vi "GUI.vi"() -> ()   [LabVIEW 2019]
uses:
  song-structure.ctl
  Project Parameters.ctl
  statemachine.ctl
  <vilib>/Platform/TimedLoop/XDataNode/timing_clust.ctl
  <vilib>/Platform/TimedLoop/XDataNode/nitl_modes.ctl
  <vilib>/Platform/TimedLoop/XDataNode/wakeup.ctl
  53cbb8c8-3a7e-4936-be36-e47a8a17bf59.vi
  <vilib>/numeric/Random Number (Range) I64.vi
  <vilib>/numeric/sub_Random U32.vi
  <vilib>/Utility/file.llb/Read Delimited Spreadsheet (string).vi
  <vilib>/platform/TimedLoop/XDataNode/XDataNode.xnode
  Windows/System32/winmm.dll
  <vilib>/Platform/TimedLoop/XDataNode/XDNodeRunTimeDep.lvlib
panel:
  out "Reaperproject folder path":path
  out "Progression":i32(knob) scale=0.0..10.0
  out "MIDI-notes":string[](array[string])
  out "Chord MIDI-values":string[][](array[string])
  out "Chord Frequencies":dbl[][][](array[numeric])
  out "Project Detail":T1
  out "Reaper Note":string
  in  "Exit":bool
  in  "Tab Control":T2(tab)
  in  "Guitarscale":bool
  out "Note 11":string
  out "Note 8":string
  out "Note 6":string
  out "Note 4":string
  out "Note 1":string
  out "Theme":string
  in  "Project name":string="Sett inn prosjektnavn her"
  out "Instruments":string[][](array[string])
  out "Special Musical Challenge":string
  out "Root":string
  out "Note 10":string
  out "Note 9":string
  out "Note 7":string
  out "Note 5":string
  out "Note 3":string
  out "Note 2":string
  out "Notes in Scale":bool[](array[boolean])
  in  "Låst BPM":i32=120
  in  "Lås BPM":bool
  out "Timesignature":string
  out "Tempo":i32
  in  "Language (H/B)":enum32{"Item 0", "Item 1"}(radio)
  in  "Initiate":bool
  out "Scale":string
  out "Key":string
  in  "Scale Categories":T3={"Minor"=TRUE, "Major"=TRUE, "Symmetric"=FALSE, "Pentatonic"=FALSE, "Bebop"=FALSE, "Blues"=FALSE, "Harmonic"=FALSE, "Exotic"=FALSE, "Misc."=FALSE}
  out "Length":string
  in  "Timesignatures":T4={"Commontime"=TRUE, "Simple"=TRUE, "Compound"=FALSE, "Complex"=FALSE}
  out "Song Structure":string[](array[string])
  in  "Reap":bool
  out "Chords":string[][](array[string])
  out "Notes":string[](array[string])
  in  "Grunntone":bool
  in  "Metronom":bool
  in  "Stop Music":bool
  in  "Ordinære\nakkorder":bool
  in  "MIDI-fil":bool
  in  "Play":bool
  in  "Create Chord Progression":bool
  out "Handler":i32
  out "Romans":string[](array[string])
  out "Chordnames":string[](array[string])
  out "Chord active":bool[](array[boolean])
  in  "Instrument":i32(listbox)
  in  "Volume":i32(slide)=99 scale=0.0..127.0
  in  "Fastest BPM":i32=170
  in  "Slowest BPM":i32=50
  in  "Song structure":T5={"Intro %"=50.0, "Bridge %"=50.0, "Solo %"=50.0, "Outro %"=50.0, "Min # Vers"=2, "Max # Vers"=5, "Min # Refreng"=2, "Max # Refreng"=4, "Measure per phrase"=4, "Phrase per part"=4} {"Outro %" format="%#_13g"; "Solo %" format="%#_13g"; "Bridge %" format="%#_13g"; "Intro %" format="%#_13g"}
  in  "CPU timing":u32=50
  in  "# instruments":i32=8
  in  "# Themes":i32=3
  out "Path of the program":path
  # "(Pick 5)"
  # "This will generate a folder! with 2 files:\n- List of chords\n- Reaper project"
  # "Available chords in the given key and scale"
  # "Chord Progression"
  # "The chord progression is generated based on the parameters from the project tab. The parameters are not altered."
  # "Settings of creation"
  # "*Not all scales work equally"
  # "Settings"
  # "I was unable to alter some of the text above without doing too much work. \"Refreng\" = Chorus, \"Vers\" = Verse. Hopefully you'll survive."
  # "About the software"
  # "Features I considered"
  # "This software was created to learn more about state machines, as well as create a software that challenges my musical/ recording skills. It's main function is to generate a musical recording challenge, by listing parameters for the user to comply to. This way the musician can focus on recording and the creative parts, instead of waiting for an idea."
  # "- Random project name\n- Jam function, without using Reaper\n-"
  # "Problems"
  # "Reaper project"
  # "At the moment the software will only have full functionality in administrative mode (Windows settings). This is only related to running a .exe-file. Avoid always having to choosing this mode by:\n1. Rightclicking the \"usic.exe\"-file.\n2. Go to settings.\n3. Open the tab \"Compatibily\".\n4.  Check the \"Run this program as administrator\" and hit OK \n\nThese names were directly translated, you experience may vary."
  # "Hvordan bruker man programmet"
  # "Under the \"Project\" tab you can generate random song parameters. Possible tempo, timesignatures and scales are selected before generating.\n\nIn the Chords tab you'll find chords that should fit the key and scale mentioned in the project tab.\n\nIn the Progression tab you can generate a chord progression that might be suitable for the given scale. Some chords and scales are more problematic. I therefore advice that you keep generating progressions and altering the settings of creation; untill you're satified with the result. The progression can then be put in stone by generating a MIDI file.\n\nThe settings tab is for thinkering with the odds of the generator."
  # "Other problems"
  # "The program crashes if you abort the creation of the reaper project folder."
  # "Musical Improv Exercise"
  # "Regler underveis"
  # "Spillet fungerer som \"ett ord om gangen eventyr\". Istedet for at hver deltaker legger til et ord, legger man til et musikalsk uttrykk.\n\n1. Den startende deltakeren starter et Reaper-prosjekt ved hjelp av dette programmet, og spiller inn ett opptak. Hvor langt opptaket er velger deltakeren selv.\n2. Prosjektet lagres og neste man får beskjed om at det er hans tur.\n3. Neste man spiller inn ett nytt opptak, og utfører punkt 2.\n\nPunkt 2 og 3 gjenntas til prosjektets krav er nådd og alle føler prosjektet er ferdig nok til miksing.\n\nStartende deltaker for i oppgave å starte miksingen, og når man føler seg ferdig blir prosjektet sendt til neste man. Dette gjentas til alle har deltatt i miksingen, miksen er nå klar for mastering.\n\nMastering fungerer på samme måte som miksing."
  # "- Bordet fanger; det vil si at man ikke kan slette tidligere endringer. Hverken sine egne innspillinger, og tillagte effekter; eller andre innspillinger. og tillagte effekter\n- Hver runde med innspilling er det mulighet for å legge effekter på spor, men ikke fjerne.\n- Det er ikke tillat å endre på prosjektparameterene oppgitt i Reaper-notatet. Altså der som genereres av startende deltaker.\n- Hver låt må ha vokal, men foruten det kan man fjerne opptil 3 instrumenter av de genererte 8.\n- Tema er opp til hver enkelt deltaker å tolke.\n- Bruker man plugins som ikke er inkludert i Reaper, må det lages et hjelpespor med effekten inebygget i sporet. Slik at man slipper plugins-en."
  # "Deling av prosjekt"
  # "Formålet"
  # "Prosjektet deles via avtalt plattform.\nHver nøye på å se over plugins."
  # "Hensikten med programmet og øvelsen er mengdetrening, eksponering og å ha det gøy. Derfor skal man ikke bruke timer på den perfekte overgangen, miksingen eller teksten. Om man ønsker en standard for musikalsk kvalitet og dybde, se til band som Bloodhound gang, Bare Egil Band,  Hurra Torpedo mm."
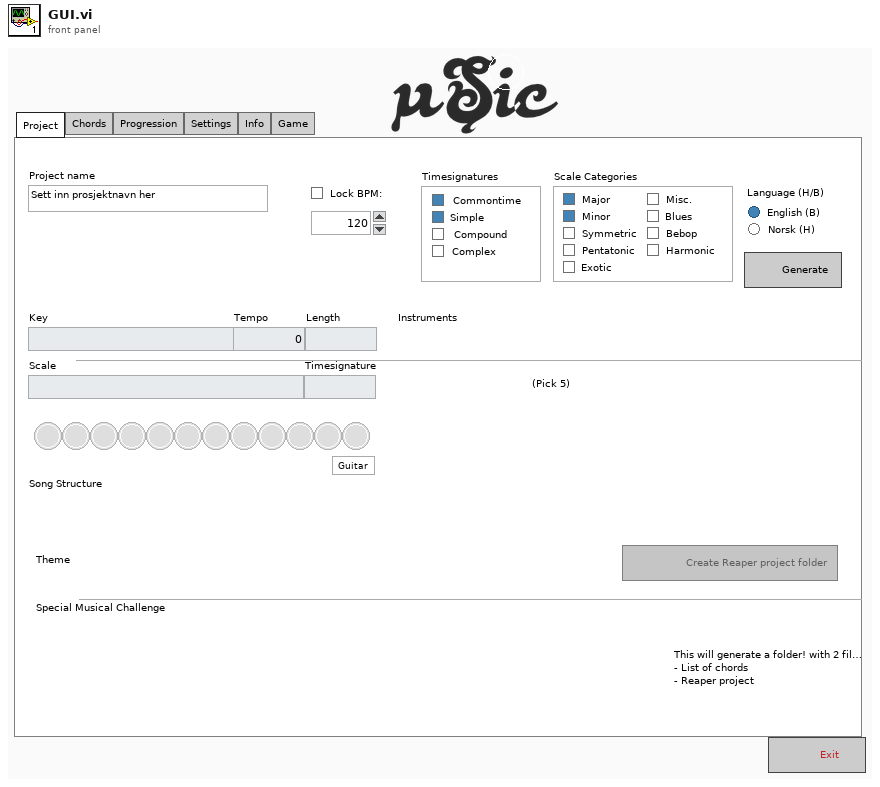
[diagram p1: front panel]
types:
  T1 = typedef "Project Parameters.ctl" = cluster{"Song Structure":string[], "Song Length":string, "Timesignature":string, "Key":string, "Scale":string, "Bpm":i32, "Tema":string, "Prosjekt tittel":string, "Challenge":string, "Instruments":string[]}
  T2 = enum32{"Project", "Chords", "Progression", "Settings", "Info", "Game"}
  T3 = cluster{"Minor":bool, "Major":bool, "Symmetric":bool, "Pentatonic":bool, "Bebop":bool, "Blues":bool, "Harmonic":bool, "Exotic":bool, "Misc.":bool}
  T4 = cluster{"Commontime":bool, "Simple":bool, "Compound":bool, "Complex":bool}
  T5 = typedef "song-structure.ctl" = cluster{"Intro %":dbl, "Bridge %":dbl, "Solo %":dbl, "Outro %":dbl, "Min # Vers":i32, "Max # Vers":i32, "Min # Refreng":i32, "Max # Refreng":i32, "Measure per phrase":i32, "Phrase per part":i32}
  T6 = typedef "statemachine.ctl" = enum16{"Boot", "Wait for Event", "Play music", "Stop music", "Shut down", "MIDI-file shutdown"}
  T7 = enum16{"open", "replace", "create", "open or create", "replace or create", "replace or create with confirmation"}
  T8 = enum8{"Enabled", "Disabled", "Disabled and Grayed Out"}
  T9 = typedef "XDNodeRunTimeDep.lvlib/timing_clust.ctl" = cluster{"Expected End [f-1]":u64, "Actual End [f-1]":u64, "Finished Late? [f-1]":bool, "Expected End [i-1]":u64, "Actual End [i-1]":u64, "Finished Late? [i-1]":bool, "Expected Start [i]":u64, "Actual Start [i]":u64, "Expected Start [f]":u64, "Actual Start [f]":u64, "Source Name":string, "Structure Name":string, "Period":i64, "Deadline":i64, "Offset":i64, "Start":i64, "Priority":i32, "Timeout":i32, "Mode":T10, "Wakeup Reason":T11, "Error":errorcluster, "Source Type":string, "Secondary Source Type":string, "Global End Time":u64, "Global Start Time":u64, "Frame Duration":u64, "Iteration Duration":u64, "Assigned CPU":i32, "I/O Scan Engine Mode":u32}
  T10 = typedef "XDNodeRunTimeDep.lvlib/nitl_modes.ctl" = enum32{"No Change", "Process missed periods, maintain original phase", "Discard missed periods, maintain original phase", "Process missed periods, ignore original phase", "Discard missed periods, ignore original phase"}
  T11 = typedef "XDNodeRunTimeDep.lvlib/wakeup.ctl" = enum32{"Normal", "Aborted", "Asynchronous wakeup", "Timing source error", "Timed loop error", "Timeout"}
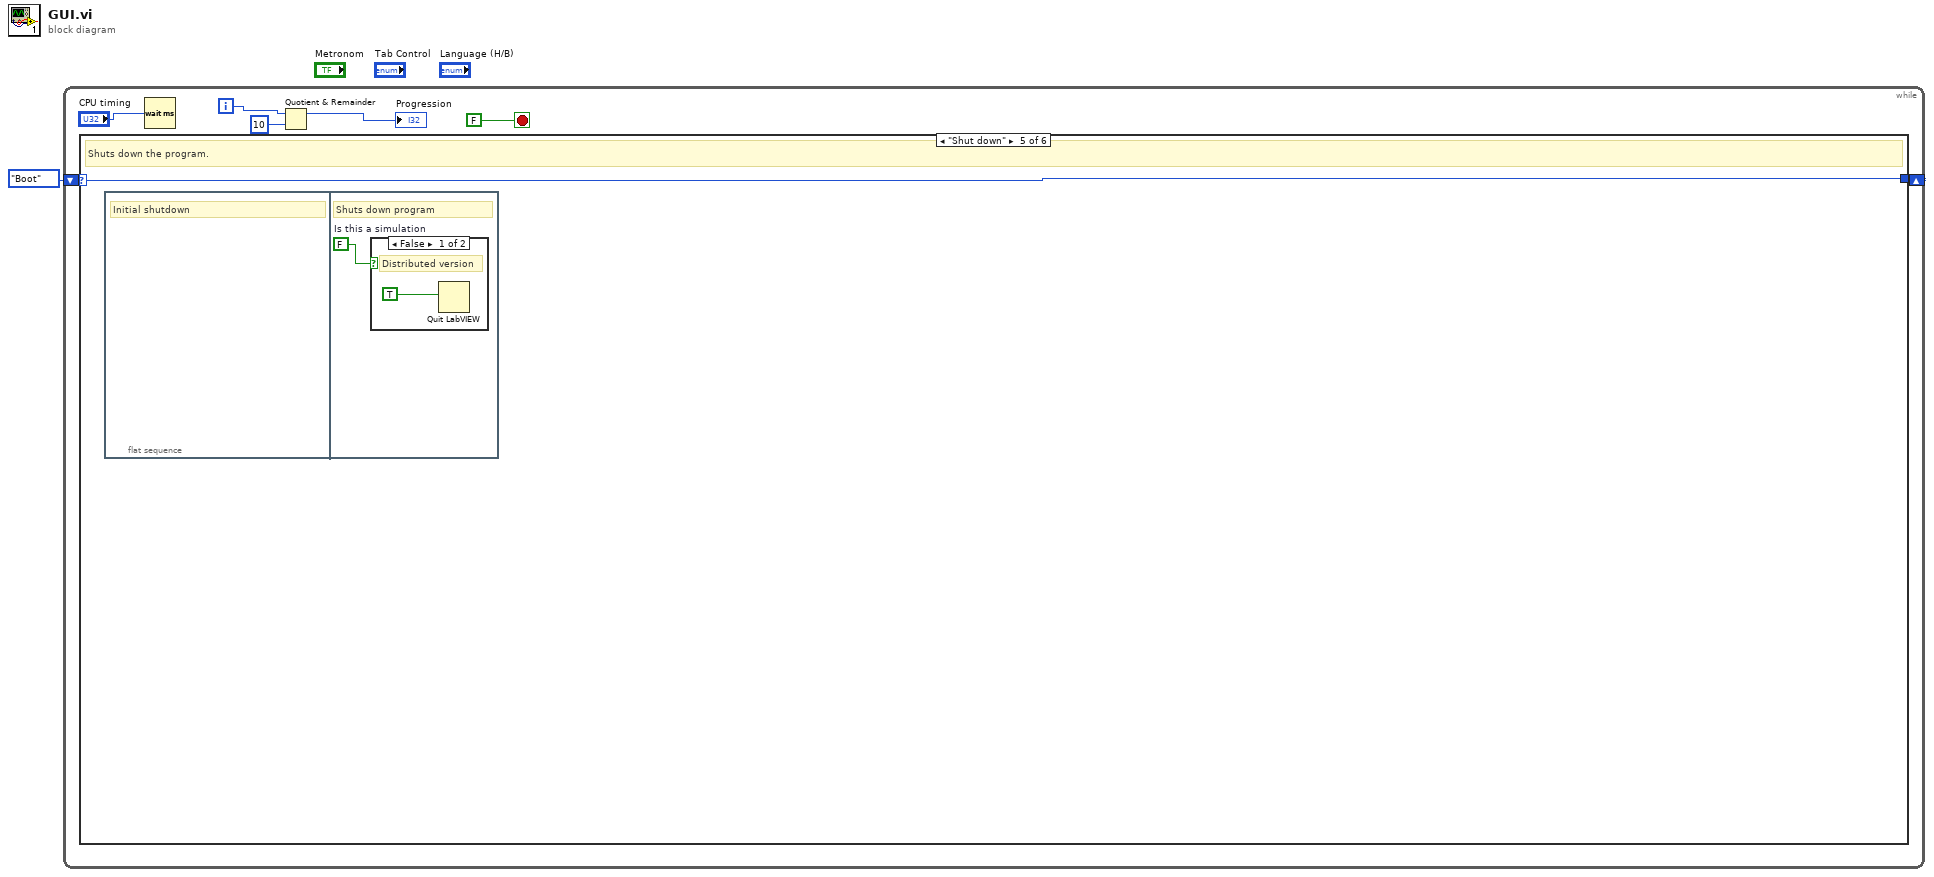
[diagram p0: block diagram]
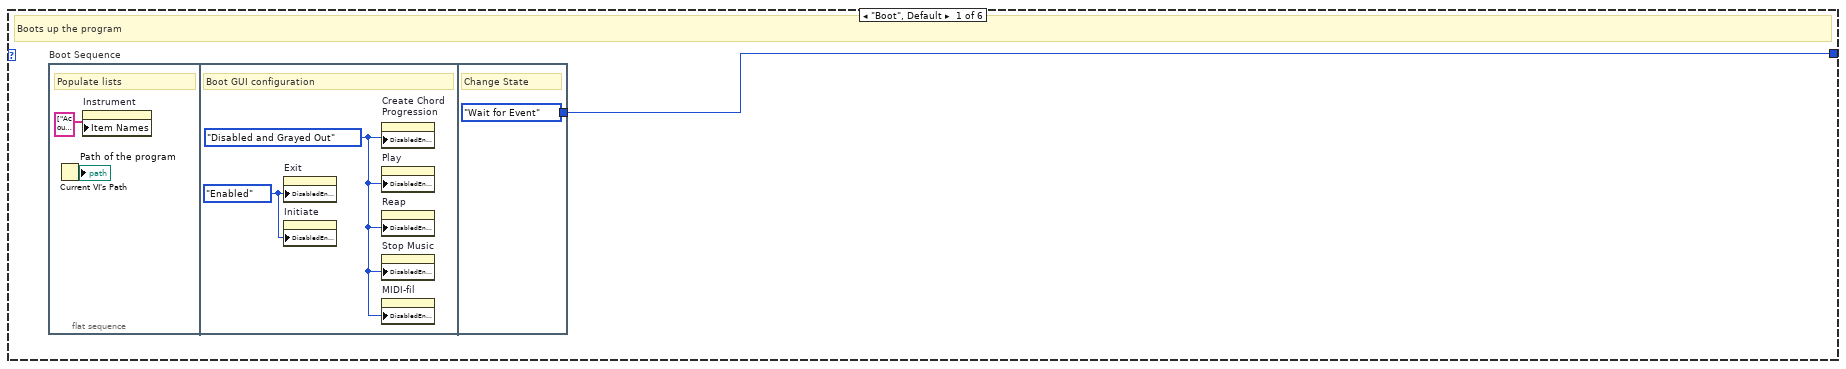
[diagram p2: hidden frame]
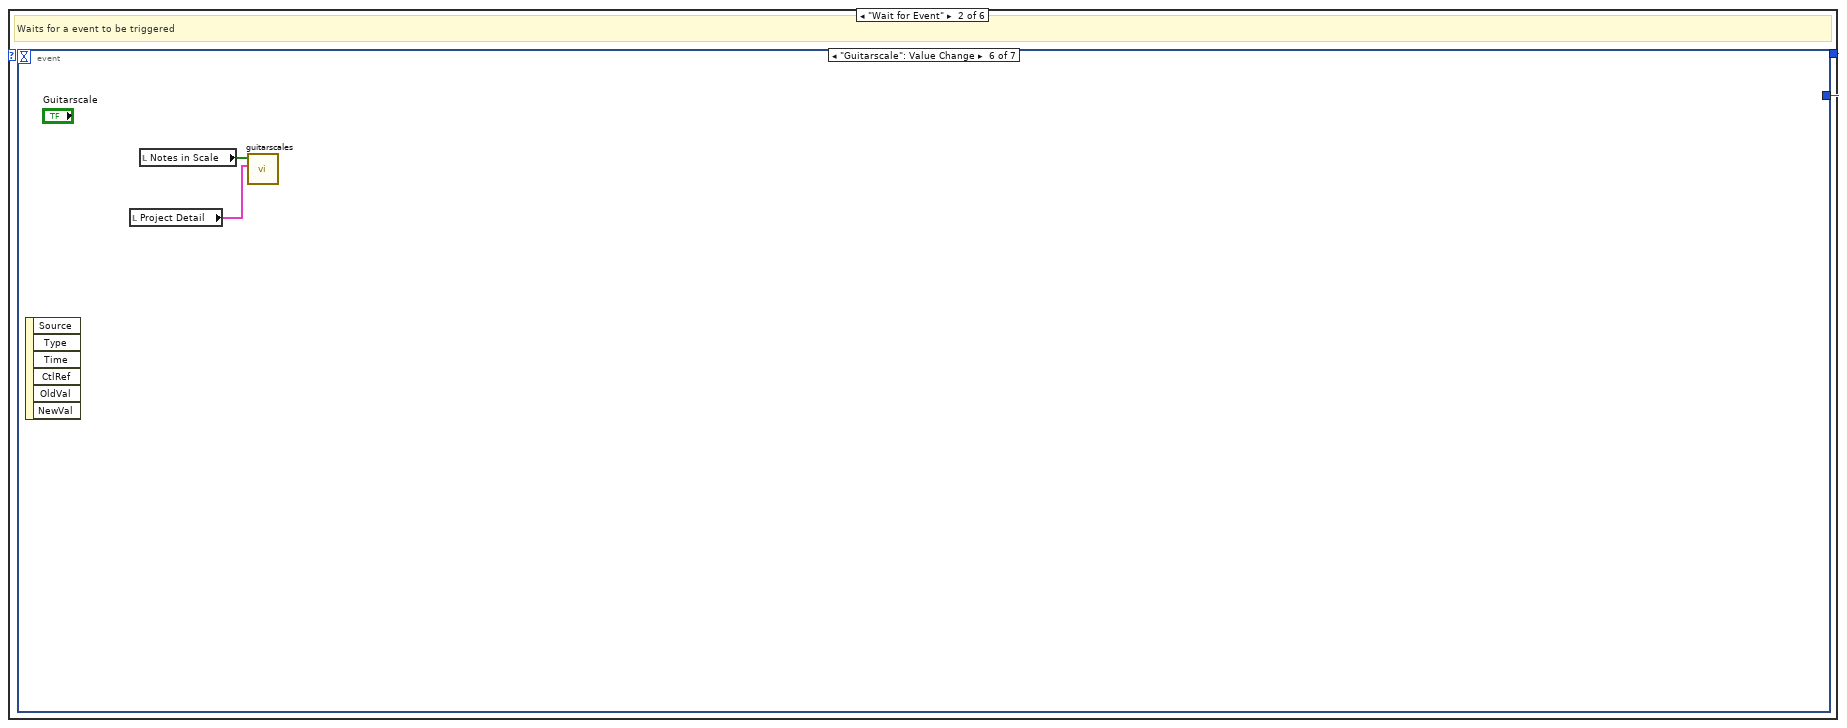
[diagram p3: hidden frame]
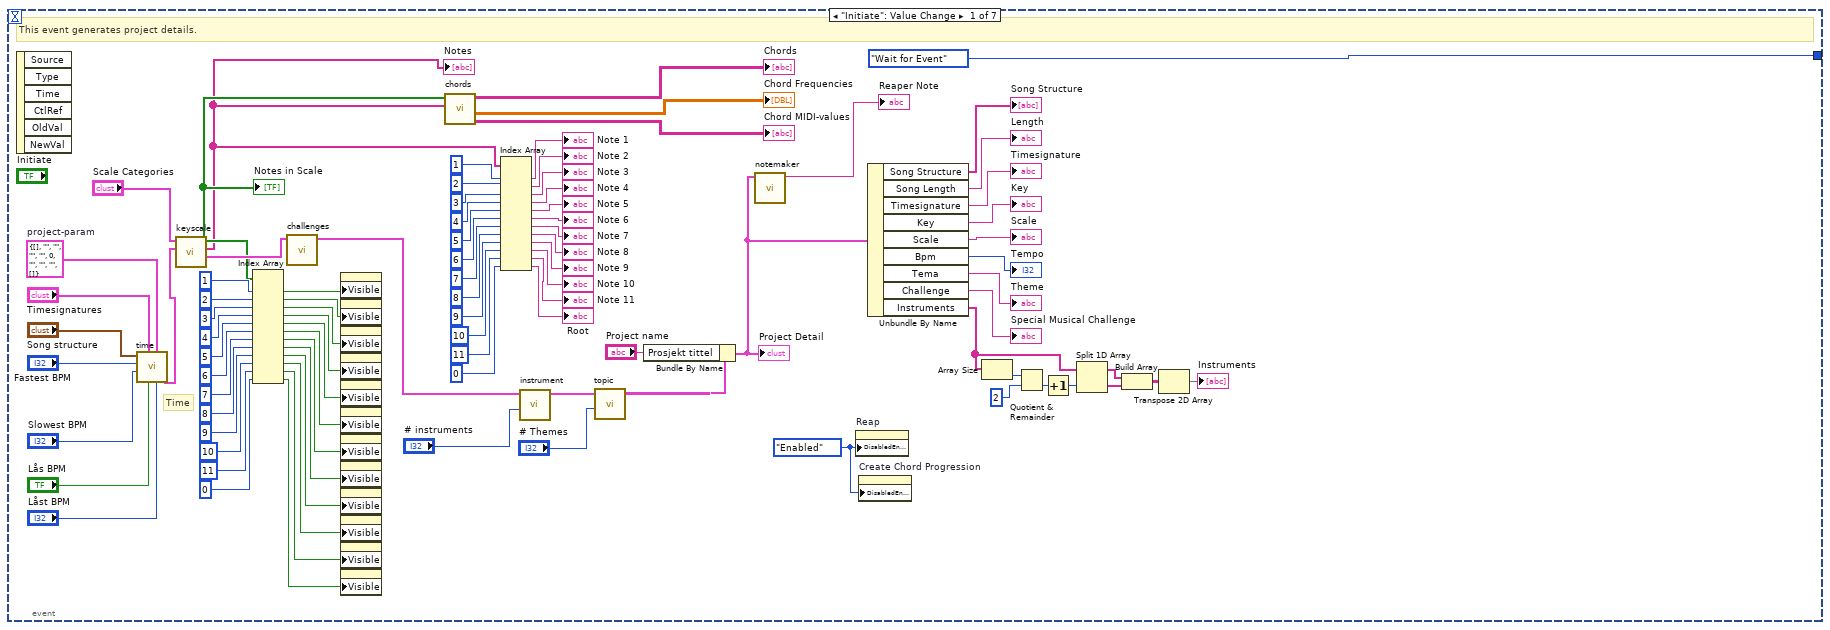
[diagram p4: hidden frame]
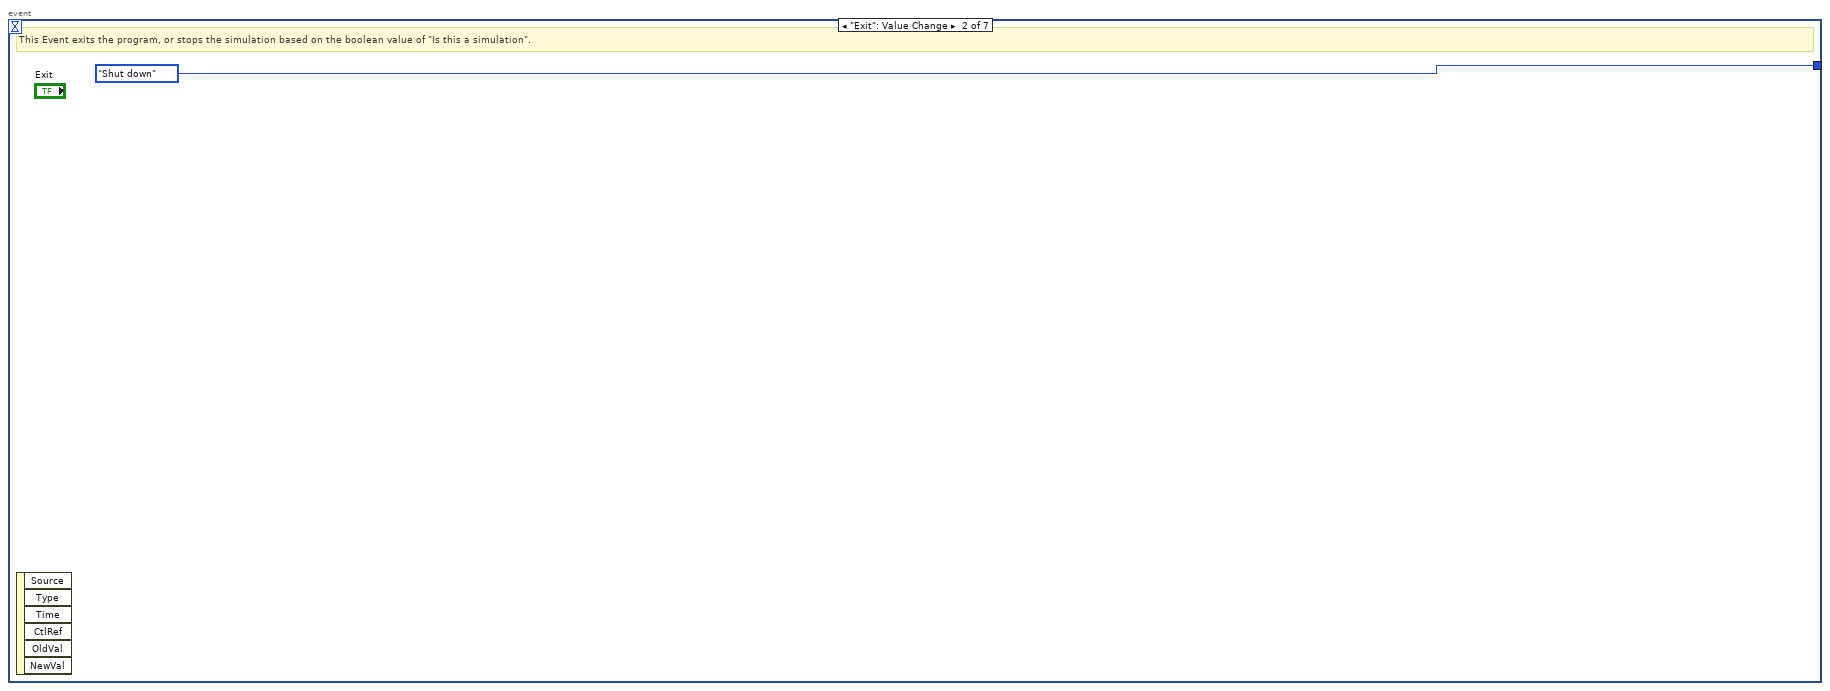
[diagram p5: hidden frame]
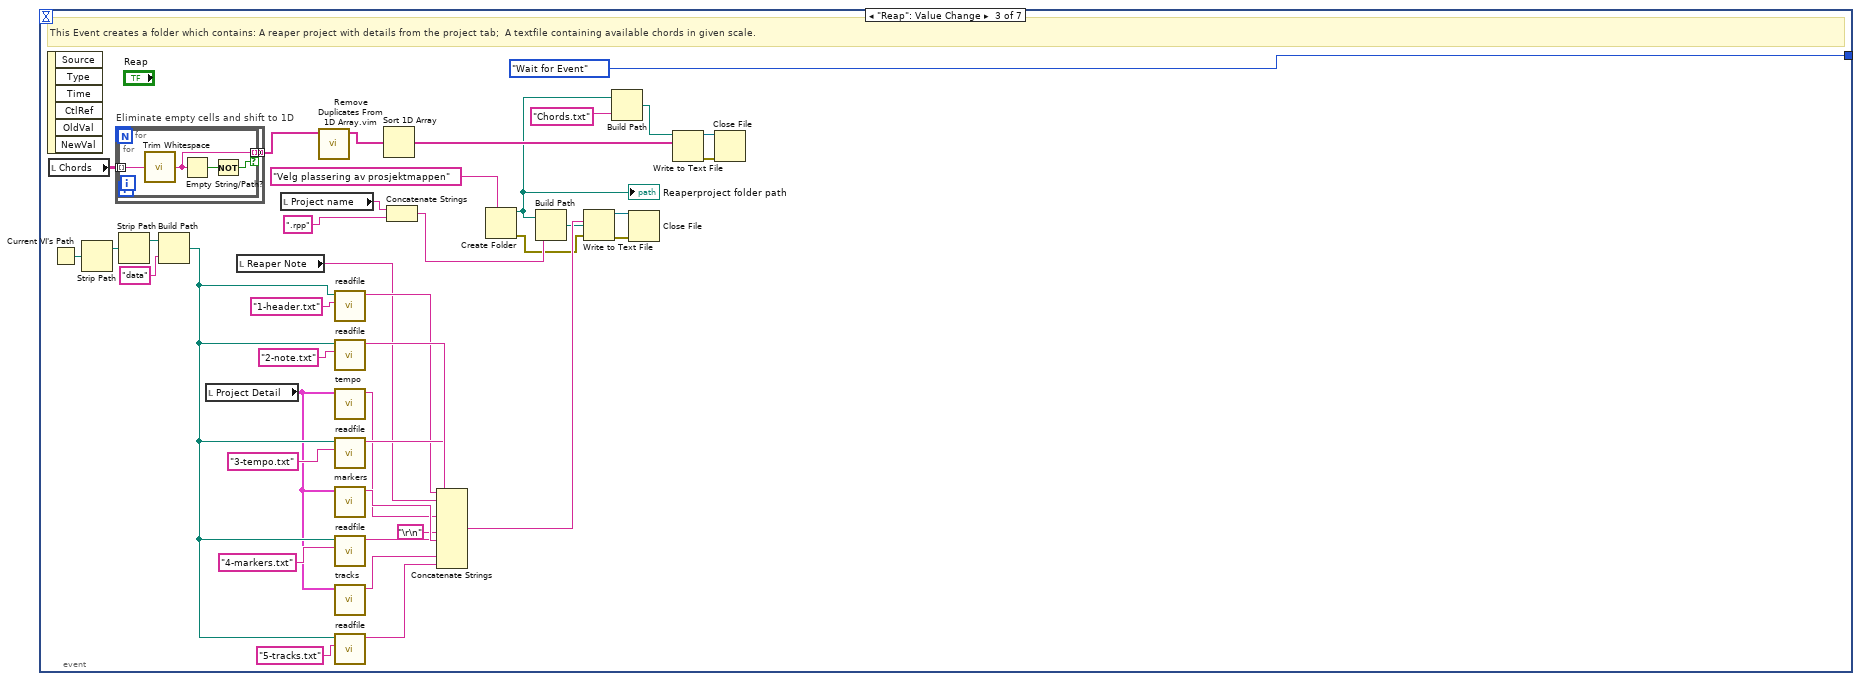
[diagram p6: hidden frame]
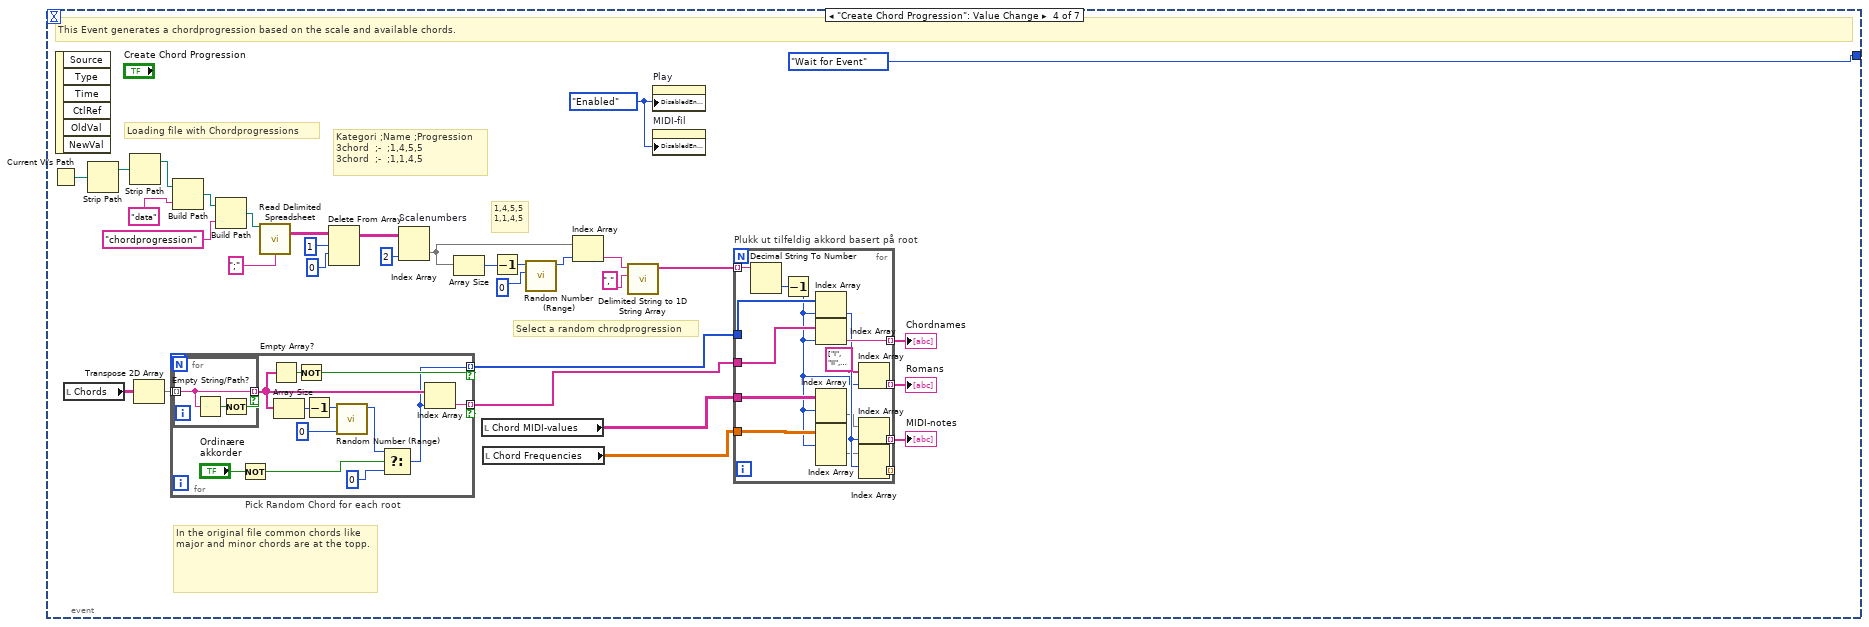
[diagram p7: hidden frame]
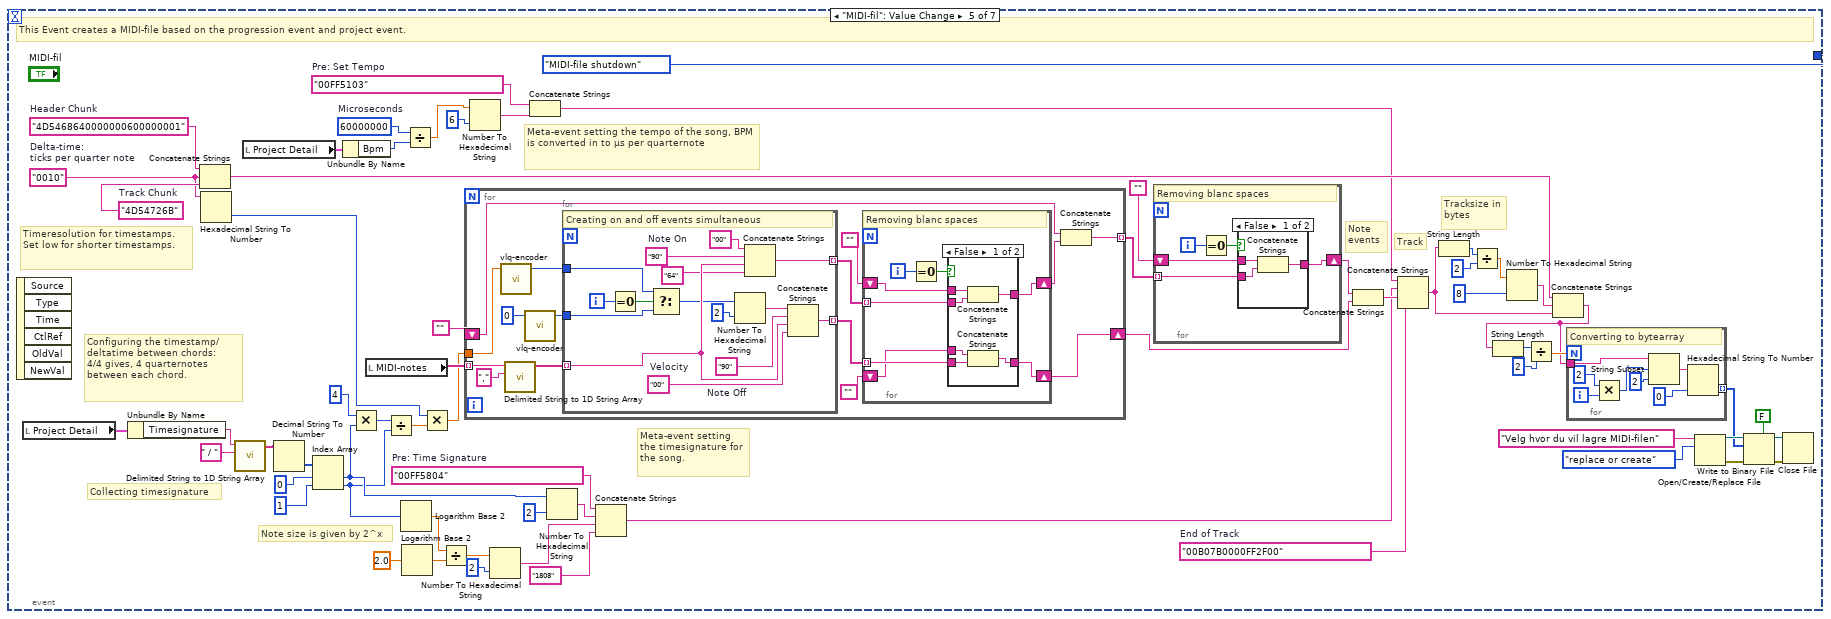
[diagram p8: hidden frame]
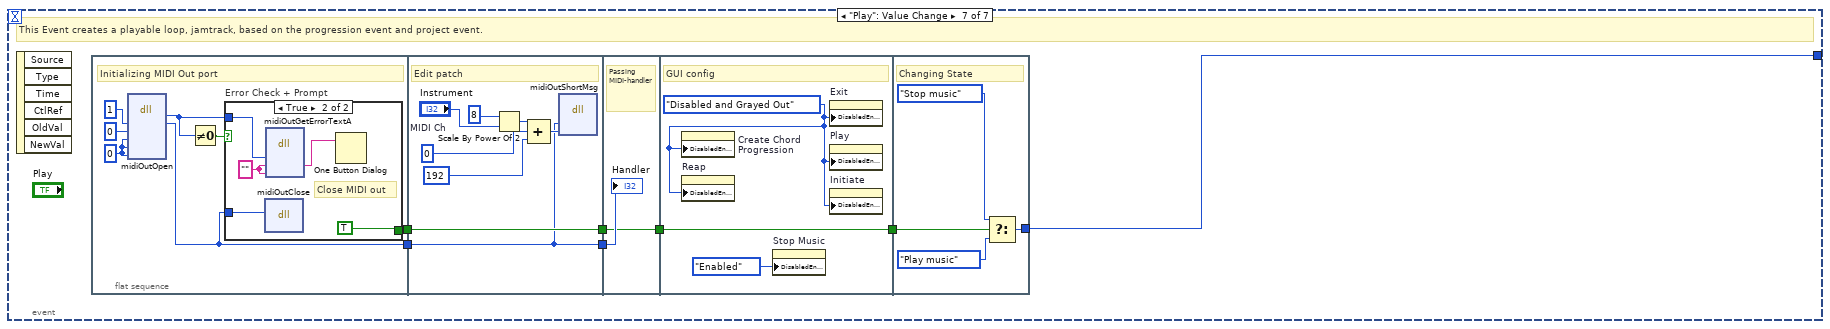
[diagram p11: hidden frame]
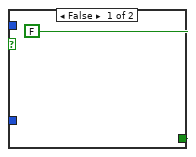
[diagram p12: hidden frame]
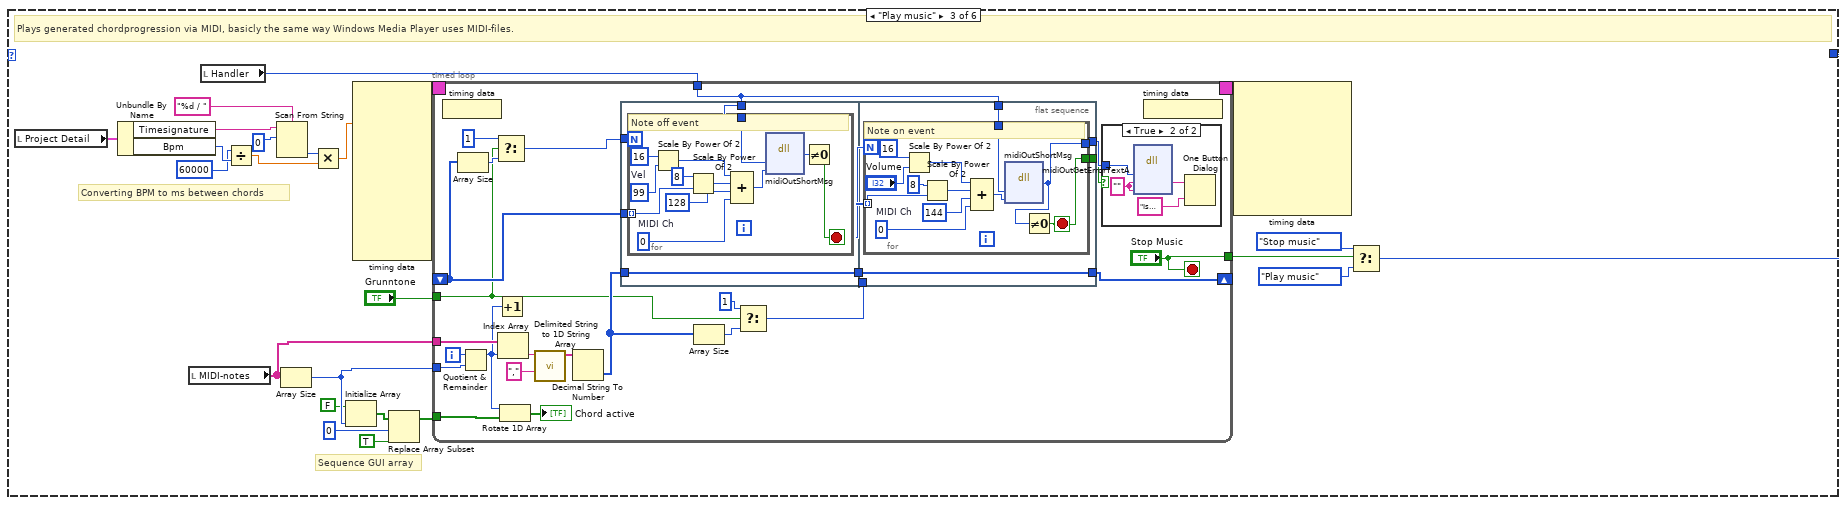
[diagram p13: hidden frame]
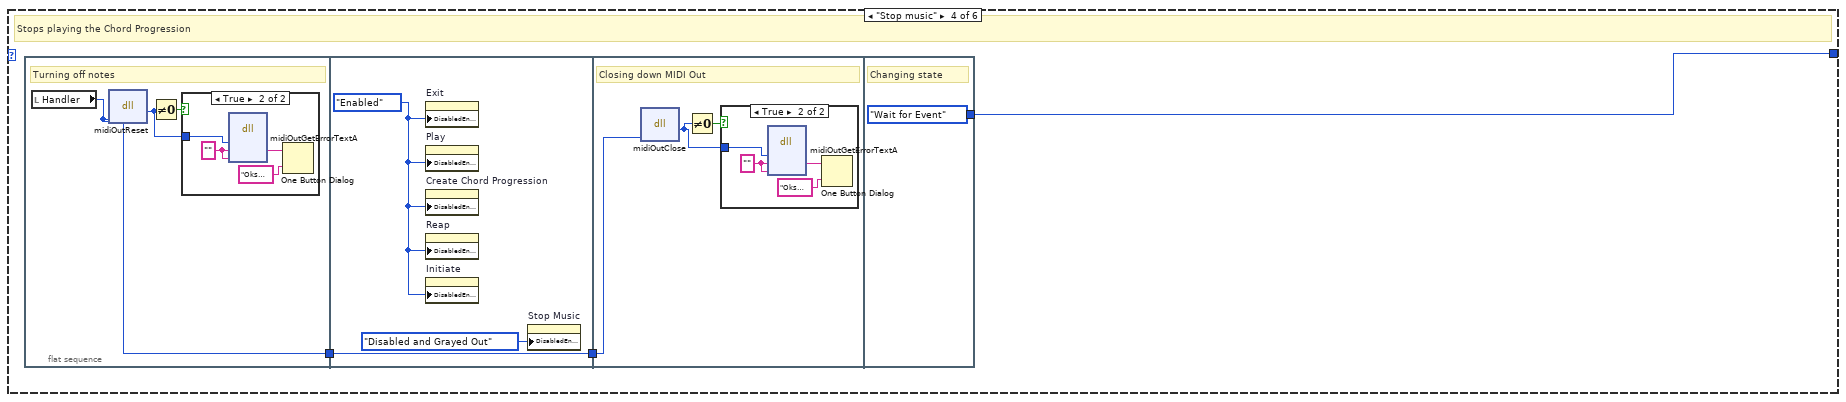
[diagram p15: hidden frame]
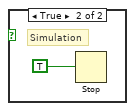
[diagram p18: hidden frame]
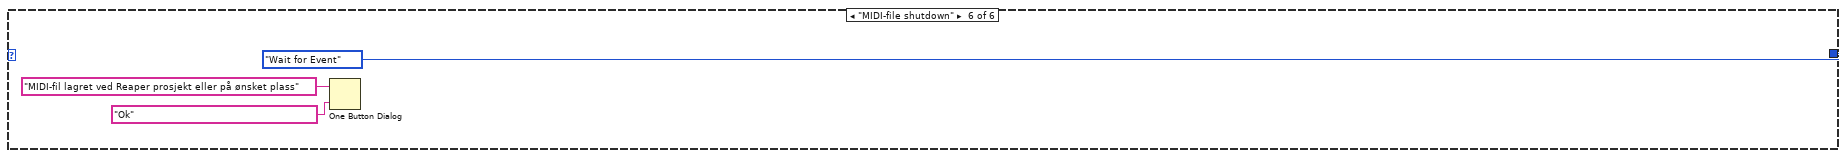
[diagram p19: hidden frame]
diagram:
  n1 = while {
    shift-right: [w2] -> _
    shift-left: statemachine."Boot" -> [w6]
    i -> [w5]
    stop <- FALSE stop-if-true
    n2 = case shown="\"Shut down\"" w6 {
      selector: w6 -> [_ _ _ _ w494 _]
      tunnel: [w9 w15 w403 w475 w494 statemachine."Wait for Event"] -> w2
      frame "Boot", Default {
        # "Boots up the program"
        n3 = flat-sequence "Boot Sequence" {
          tunnel: [statemachine."Wait for Event"] -> w9
          frame #0 {
            # "Populate lists"
            n4 = Current VI's Path() -> (path=→"Path of the program":path)
            n5 = property on="Instrument" class="LstBox (strict)"("Item Names"=string[] ["Acoustic Grand ", "Bright Acoustic ", "Electric Grand ", "Honky-tonk ", "Electric Piano I ", "Electric Piano 2 ", "Harpsichord ", "Clav ", "Perc Celesta ", "Perc Glockenspiel ", "Perc Music Box ", "Perc Vibraphone ", "Perc Marimba ", "Perc Xylophone ", "Perc Tubular Bells ", "perc Dulcimer ", "Drawbar Organ ", "Percussive Organ ", "Rock Organ ", "Church Organ ", "Reed Organ ", "Accordian ", "Harmonica ", "Tango Accordian ", "Acoustic Guitar (nylon) ", "Acoustic Guitar (steel) ", "Electric Guitar (jazz) ", "Electric Guitar (clean) ", "Electric Guitar (muted) ", "Overdriven Guitar ", "Distortion Guitar ", "Guitar Harmonics ", "Acoustic Bass ", "Electric Bass (finger) ", "Electric Bass (pick) ", "Fretless Bass ", "Slap Bass 1 ", "Slap Bass 2 ", "Synth Bass I ", "Synth Bass 2 ", "Violin ", "Viola ", "Cello ", "Contrabass ", "Tremolo Strings ", "Pizzicato Strings ", "Orchestral Strings ", "Timpani ", "String Ensemble 1 ", "String Ensemble 2 ", "Synth Strings I ", "Synth Strings 2 ", "Choir Aahs ", "Voice Oohs ", "Synth Voice ", "Orchestra Hit ", "Trumpet ", "Trombone ", "Tuba ", "Muted Trumpet ", "French Horn ", "Brass Section ", "Synth Brass I ", "Synth Brass 2 ", "Soprano Saxophone ", "Alto Saxophone ", "Tenor Saxophone ", "Baritone Saxophone ", "Oboe ", "English Horn ", "Bassoon ", "Clarinet ", "Piccolo ", "Flute ", "Recorder ", "Pan Flute ", "Blown Bottle ", "Shakuhachi ", "Whistle ", "Ocarina ", "Lead Lead 1 (square) ", "Lead Lead 2 (sawtooth) ", "Lead Lead 3 (calliope) ", "Lead Lead 4 (chiff) ", "Lead Lead 5 (charang) ", "Lead Lead 6 (voice) ", "Lead Lead 7 (fifths) ", "Lead Lead 8 (bass + lead) ", "Pad Pad 1 (new age) ", "Pad Pad 2 (warm) ", "Pad Pad 3 (polysynth) ", "Pad Pad 4 (choir) ", "Pad Pad 5 (bowed) ", "Pad Pad 6 (metallic) ", "Pad Pad 7 (halo) ", "Pad Pad 8 (sweep) ", "FX FX 1 (rain) ", "FX FX2 (soundtrack) ", "FX FX 3 (crystal) ", "FX FX 4 (atmosphere) ", "FX FX 5 (brightness) ", "FX FX 6 (goblins) ", "FX FX 7 (echoes) ", "FX FX 8 (sci-fi) ", "Sitar ", "Banjo ", "Shamisen ", "Koto ", "Kalimba ", "Bagpipe ", "Fiddle ", "Shanai ", "Tinkle Bell ", "Agogo ", "Steel Drums ", "Woodblock ", "Taiko Drum ", "Melodic Tom ", "Synth Drum ", "Reverse Cymbal ", "FX Guitar Fret Noise ", "FX Breathing Noise ", "FX Seashore ", "FX Bird Tweet ", "FX Telephone Ring ", "FX Helicopter ", "FX Applause ", "FX Gunshot "]) -> ()  [unwired: 2 in, 2 out]
          }
          frame #1 {
            w13 = T8."Enabled" ("Disabled")
            w12 = T8."Disabled and Grayed Out" ("Disabled")
            # "Boot GUI configuration"
            n6 = property on="Exit" class="Bool"("DisabledEnum"=w13) -> ()  [unwired: 2 in, 2 out]
            n7 = property on="Initiate" class="Bool"("DisabledEnum"=w13) -> ()  [unwired: 2 in, 2 out]
            n8 = property on="Create Chord\nProgression" class="Bool"("DisabledEnum"=w12) -> ()  [unwired: 2 in, 2 out]
            n9 = property on="Play" class="Bool"("DisabledEnum"=w12) -> ()  [unwired: 2 in, 2 out]
            n10 = property on="Reap" class="Bool"("DisabledEnum"=w12) -> ()  [unwired: 2 in, 2 out]
            n11 = property on="Stop Music" class="Bool"("DisabledEnum"=w12) -> ()  [unwired: 2 in, 2 out]
            n12 = property on="MIDI-fil" class="Bool"("DisabledEnum"=w12) -> ()  [unwired: 2 in, 2 out]
          }
          frame #2 {
            # "Change State"
          }
        }
      }
      frame "Wait for Event" {
        # "Waits for a event to be triggered"
        n13 = event shown="[5] \"Guitarscale\": Value Change" {
          selector: _ -> [_ _ _ _ _ _ _]
          dyn-events: _ -> [_ _ _ _ _ _ _]
          timeout: _ -> [_ _ _ _ _ _ _]
          tunnel: [statemachine."Wait for Event" statemachine."Shut down" statemachine."Wait for Event" statemachine."Wait for Event" statemachine."MIDI-file shutdown" _ w351] -> w15
          event "Initiate": Value Change {
            w16 = T8."Enabled" ("Disabled")
            w50 = T1 {"Song Structure"=[], "Song Length"="", "Timesignature"="", "Key"="", "Scale"="", "Bpm"=0, "Tema"="", "Prosjekt tittel"="", "Challenge"="", "Instruments"=[]}  # project-param
            # "Time"
            # "This event generates project details."
            n14 = event-data() -> ()  [unwired: 1 in, 6 out]
            n15 = call "time.vi"("Låst BPM"="Låst BPM", "project-param in"=w50, "Lås BPM"="Lås BPM", "Time Signatures"="Timesignatures", "Lower BPM"="Slowest BPM", "Upper BPM"="Fastest BPM", "Song structure"="Song structure") -> ("project-param out"=w49:T1)  [unwired: 4 in]
            n16 = call "keyscale.vi"("project-param in"=w49, "Scales"="Scale Categories") -> ("project-param out 2"=w40:T1, "Array"=w21:string[], "Scale Notes"=w22:bool[])  [unwired: 7 in]
            "Notes in Scale" <- w22
            "Notes" <- w21
            n17 = Index Array(array=w22, index #1=1 ("index"), index #2=2 ("index"), index #3=3 ("index"), index #4=4 ("index"), index #5=5 ("index"), index #6=6 ("index"), index #7=7 ("index"), index #8=8 ("index"), index #9=9 ("index"), index #10=10 ("index"), index #11=11 ("index"), index #12=0 ("index")) -> (element #1=w98:bool, element #2=w63:bool, element #3=w62:bool, element #4=w61:bool, element #5=w60:bool, element #6=w59:bool, element #7=w58:bool, element #8=w57:bool, element #9=w56:bool, element #10=w55:bool, element #11=w54:bool, element #12=w53:bool)
            n18 = call "challenges.vi"("project-param out 3"=w40) -> ("project-param out 2"=w39:T1)  [unwired: 10 in]
            n19 = property on="Note 1" class="Str"("Visible"=w98) -> ()  [unwired: 2 in, 2 out]
            n20 = property on="Note 2" class="Str"("Visible"=w63) -> ()  [unwired: 2 in, 2 out]
            n21 = property on="Note 3" class="Str"("Visible"=w62) -> ()  [unwired: 2 in, 2 out]
            n22 = property on="Note 4" class="Str"("Visible"=w61) -> ()  [unwired: 2 in, 2 out]
            n23 = property on="Note 5" class="Str"("Visible"=w60) -> ()  [unwired: 2 in, 2 out]
            n24 = property on="Note 6" class="Str"("Visible"=w59) -> ()  [unwired: 2 in, 2 out]
            n25 = property on="Note 7" class="Str"("Visible"=w58) -> ()  [unwired: 2 in, 2 out]
            n26 = property on="Note 8" class="Str"("Visible"=w57) -> ()  [unwired: 2 in, 2 out]
            n27 = property on="Note 9" class="Str"("Visible"=w56) -> ()  [unwired: 2 in, 2 out]
            n28 = property on="Note 10" class="Str"("Visible"=w55) -> ()  [unwired: 2 in, 2 out]
            n29 = property on="Note 11" class="Str"("Visible"=w54) -> ()  [unwired: 2 in, 2 out]
            n30 = property on="Root" class="Str"("Visible"=w53) -> ()  [unwired: 2 in, 2 out]
            n31 = call "chords.vi"("Notenames"=w21, "Notes in Scale"=w22) -> ("MIDI-values"=→"Chord MIDI-values":string[][], "Chord Frequencies"=→"Chord Frequencies":dbl[][][], "Chords"=→"Chords":string[][])  [unwired: 7 in]
            n32 = Index Array(array=w21, index #1=1 ("index"), index #2=2 ("index"), index #3=3 ("index"), index #4=4 ("index"), index #5=5 ("index"), index #6=6 ("index"), index #7=7 ("index"), index #8=8 ("index"), index #9=9 ("index"), index #10=10 ("index"), index #11=11 ("index"), index #12=0 ("index")) -> (element #1=→"Note 1":string, element #2=→"Note 2":string, element #3=→"Note 3":string, element #4=→"Note 4":string, element #5=→"Note 5":string, element #6=→"Note 6":string, element #7=→"Note 7":string, element #8=→"Note 8":string, element #9=→"Note 9":string, element #10=→"Note 10":string, element #11=→"Note 11":string, element #12=→"Root":string)
            n33 = call "instrument.vi"("Amount of Instruments"="# instruments", "project-param in"=w39) -> ("project-param out 3"=w37:T1)  [unwired: 9 in]
            n34 = call "topic.vi"("Amount of topics"="# Themes", "project-param out 4"=w37) -> ("project-param out 3"=w36:T1)  [unwired: 9 in]
            n35 = Bundle By Name(cluster=w36, "Prosjekt tittel"="Project name") -> (w20:T1)
            "Project Detail" <- w20
            n36 = call "notemaker.vi"("project-param in"=w20) -> ("Reaper Note"=→"Reaper Note":string)  [unwired: 10 in]
            n37 = property on="Reap" class="Bool"("DisabledEnum"=w16) -> ()  [unwired: 2 in, 2 out]
            n38 = property on="Create Chord Progression" class="Bool"("DisabledEnum"=w16) -> ()  [unwired: 2 in, 2 out]
            n39 = Unbundle By Name(w20) -> ("Song Structure"=→"Song Structure":string[], "Song Length"=→"Length":string, "Timesignature"=→"Timesignature":string, "Key"=→"Key":string, "Scale"=→"Scale":string, "Bpm"=→"Tempo":i32, "Tema"=→"Theme":string, "Challenge"=→"Special Musical Challenge":string, "Instruments"=w32:string[])
            n40 = Array Size(array=w32) -> (size(s)=w31:i32)
            n41 = Quotient & Remainder(x=w31, y=2) -> (floor(x/y)=w29:i32)  [unwired: 1 out]
            n42 = Increment(x=w29) -> (x+1=w28:i32)
            n43 = Split 1D Array(array=w32, index=w28) -> (first subarray=w27:string[], second subarray=w26:string[])
            n44 = Build Array(w27, w26) -> (w25:string[][])
            n45 = Transpose 2D Array(2D array=w25) -> (transposed array=→"Instruments":string[][])
          }
          event "Exit": Value Change {
            # "This Event exits the program, or stops the simulation based on the boolean value of \"Is this a simulation\"."
            n46 = event-data() -> ()  [unwired: 1 in, 6 out]
          }
          event "Reap": Value Change {
            # "This Event creates a folder which contains: A reaper project with details from the project tab;  A textfile containing available chords in given scale."
            n47 = event-data() -> ()  [unwired: 1 in, 6 out]
            n48 = local read "Chords"() -> (w121:string[][])
            n49 = Current VI's Path() -> (path=w146:path)
            n50 = Strip Path ("Relative Path")(path=w146) -> (stripped path=w126:path)  [unwired: 1 out]
            n51 = for "Eliminate empty cells and shift to 1D" {
              tunnel: w121 -> [w148] mode=indexing
              tunnel: [w147] -> w123 mode=concatenating
              n52 = for {
                tunnel: w148 -> [w152] mode=indexing
                tunnel: [w151] -> w147 mode=indexing if=w149
                n53 = call <vilib>:"Trim Whitespace.vi"("string"=w152) -> ("trimmed string"=w151:string)  [unwired: 1 in]
                n54 = Empty String/Path?(string/path=w151) -> (empty?=w150:bool)
                n55 = Not(x=w150) -> (.not. x?=w149:bool)
              }
            }
            n56 = Strip Path ("Relative Path")(path=w126) -> (stripped path=w125:path)  [unwired: 1 out]
            n57 = Build Path ("datafiles")(base path=w125, name or relative path="data") -> (appended path=w129:path)
            n58 = local read "Project Detail"() -> (w120:T1)
            n59 = local read "Reaper Note"() -> (w124:string)
            n60 = local read "Project name"() -> (w109:string)
            n61 = call "Remove Duplicates From 1D Array.vim"("array"=w123) -> ("array with duplicates removed"=w122:string[])  [unwired: 10 in]
            n62 = call "readfile.vi"("name or relative path"="1-header.txt", "Relative Path"=w129) -> ("String"=w137:string)  [unwired: 9 in]
            n63 = call "readfile.vi"("name or relative path"="2-note.txt", "Relative Path"=w129) -> ("String"=w143:string)  [unwired: 9 in]
            n64 = call "tempo.vi"("project-param out 3"=w120) -> ("String"=w131:string)  [unwired: 10 in]
            n65 = call "readfile.vi"("name or relative path"="3-tempo.txt", "Relative Path"=w129) -> ("String"=w138:string)  [unwired: 9 in]
            n66 = call "markers.vi"("project-param in"=w120) -> ("delimited string"=w134:string)  [unwired: 10 in]
            n67 = call "readfile.vi"("name or relative path"="4-markers.txt", "Relative Path"=w129) -> ("String"=w133:string)  [unwired: 9 in]
            n68 = call "tracks.vi"("project-param out 3"=w120) -> ("delimited string"=w127:string)  [unwired: 10 in]
            n69 = call "readfile.vi"("name or relative path"="5-tracks.txt", "Relative Path"=w129) -> ("String"=w128:string)  [unwired: 9 in]
            n70 = Sort 1D Array(array=w122) -> (sorted array=w111:string[])
            n71 = Concatenate Strings(w109, ".rpp" ("string")) -> (w117:string)
            n72 = Concatenate Strings(w137, w124, w143, w131, w138, "\r\n", w134, w133, w127, w128) -> (w140:string)
            n73 = Create Folder(prompt (Create Folder)="Velg plassering av prosjektmappen") -> (created path=w107:path, error out=w110:errorcluster)  [unwired: 2 in, 1 out]
            "Reaperproject folder path" <- w107
            n74 = Build Path ("datafiles")(base path=w107, name or relative path=w117) -> (appended path=w116:path)
            n75 = Write to Text File(file (use dialog)=w116, text=w140, error in=w110) -> (refnum out=w141:refnum<file>, error out=w142:errorcluster)  [unwired: 1 in, 1 out]
            n76 = Build Path ("datafiles")(base path=w107, name or relative path="Chords.txt") -> (appended path=w115:path)
            n77 = Close File(refnum=w141, error in=w142) -> ()  [unwired: 2 out]
            n78 = Write to Text File(file (use dialog)=w115, text=w111) -> (refnum out=w114:refnum<file>, error out=w113:errorcluster)  [unwired: 2 in, 1 out]
            n79 = Close File(refnum=w114, error in=w113) -> ()  [unwired: 2 out]
          }
          event "Create Chord Progression": Value Change {
            w153 = T8."Enabled" ("Disabled")
            # "In the original file common chords like major and minor chords are at the topp."
            # "1,4,5,5\n1,1,4,5"
            # "Kategori\t;Name\t;Progression\n3chord\t\t;-\t\t;1,4,5,5\n3chord\t\t;-\t\t;1,1,4,5"
            # "Select a random chrodprogression"
            # "Loading file with Chordprogressions"
            # "This Event generates a chordprogression based on the scale and available chords."
            n80 = Current VI's Path() -> (path=w184:path)
            n81 = event-data() -> ()  [unwired: 1 in, 6 out]
            n82 = local read "Chords"() -> (w167:string[][])
            n83 = Strip Path ("Relative Path")(path=w184) -> (stripped path=w182:path)  [unwired: 1 out]
            n84 = Strip Path ("Relative Path")(path=w182) -> (stripped path=w181:path)  [unwired: 1 out]
            n85 = Transpose 2D Array(2D array=w167) -> (transposed array=w166:string[][])
            n86 = for "Pick Random Chord for each root" {
              tunnel: w166 -> [w212] mode=indexing
              tunnel: [w206] -> w165 mode=indexing if=w205
              tunnel: [w201] -> w160 mode=indexing if=w205
              n87 = for {
                tunnel: [w215] -> w207 mode=indexing if=w213
                tunnel: w212 -> [w215] mode=indexing
                n88 = Empty String/Path?(string/path=w215) -> (empty?=w214:bool)
                n89 = Not(x=w214) -> (.not. x?=w213:bool)
              }
              n90 = Not(x="Ordinære\nakkorder") -> (.not. x?=w200:bool)
              n91 = Empty Array?(array=w207) -> (empty?=w211:bool)
              n92 = Array Size(array=w207) -> (size(s)=w210:i32)
              n93 = Not(x=w211) -> (.not. x?=w205:bool)
              n94 = Decrement(x=w210) -> (x-1=w208:i32)
              n95 = call-poly <vilib>:"Random Number (Range).vi"("lower bound (-100)"=i64 0, "upper bound (100)"=w208) -> ("number"=w204:i64)  [unwired: 9 in]
              n96 = Select(t=w204, s=w200, f=0) -> (s? t:f=w201:i64)
              n97 = Index Array(array=w207, index=w201) -> (element=w206:string)
            }
            n98 = Build Path ("datafiles")(base path=w181, name or relative path="data") -> (appended path=w178:path)
            n99 = Build Path(base path=w178, name or relative path="chordprogression") -> (appended path=w179:path)
            n100 = call-poly <vilib>:"Read Delimited Spreadsheet.vi"("file path (dialog if empty)"=w179, "delimiter (\\t)"=";" ("delimiter (\\t)")) -> ("all rows"=w172:string[][])  [unwired: 8 in, 5 out]
            n101 = Delete From Array(array=w172, length=1, index (row)=0) -> (array with subset deleted=w170:string[][])  [unwired: 1 in, 1 out]
            n102 = Index Array "Scalenumbers"(array=w170, index (col)=2 ("index (row)")) -> (element=w169:string[])  [unwired: 1 in]
            n103 = Array Size(array=w169) -> (size(s)=w177:i32)
            n104 = local read "Chord MIDI-values"() -> (w159:string[][])
            n105 = local read "Chord Frequencies"() -> (w158:dbl[][][])
            n106 = Decrement(x=w177) -> (x-1=w164:i32)
            n107 = call-poly <vilib>:"Random Number (Range).vi"("lower bound (-100)"=i64 0, "upper bound (100)"=w164) -> ("number"=w175:i64)  [unwired: 9 in]
            n108 = Index Array(array=w169, index=w175) -> (element=w162:string)
            n109 = call <vilib>:"Delimited String to 1D String Array.vi"("delimiter"=",", "delimited string"=w162) -> ("string array"=w161:string[])  [unwired: 9 in]
            n110 = property on="Play" class="Bool"("DisabledEnum"=w153) -> ()  [unwired: 2 in, 2 out]
            n111 = property on="MIDI-fil" class="Bool"("DisabledEnum"=w153) -> ()  [unwired: 2 in, 2 out]
            n112 = for "Plukk ut tilfeldig akkord basert på root" {
              tunnel: w161 -> [w199] mode=indexing
              tunnel: w165 -> [w198]
              tunnel: [w197] -> w155 mode=indexing
              tunnel: w160 -> [w195]
              tunnel: w159 -> [w193]
              tunnel: w158 -> [w194]
              tunnel: [w189] -> w157 mode=indexing
              tunnel: [w188] -> _ mode=indexing
              tunnel: [w185] -> w154 mode=indexing
              n113 = Decimal String To Number(string=w199) -> (number=w196:i32)  [unwired: 2 in, 1 out]
              n114 = Decrement(x=w196) -> (x-1=w187:i32)
              n115 = Index Array(array=w195, index=w187) -> (element=w192:i64)
              n116 = Index Array(array=w198, index=w187) -> (element=w197:string)
              n117 = Index Array(array=w193, index (row)=w187) -> (element=w190:string[])  [unwired: 1 in]
              n118 = Index Array(array=w194, index (dim 0)=w187) -> (element=w191:dbl[][])  [unwired: 2 in]
              n119 = Index Array(array=string[] ["I", "II", "III", "IV", "V", "VI", "VII", "VIII", "IX", "X", "XI"], index=w187) -> (element=w185:string)
              n120 = Index Array(array=w190, index=w192) -> (element=w189:string)
              n121 = Index Array(array=w191, index (row)=w192) -> (element=w188:dbl[])  [unwired: 1 in]
            }
            "MIDI-notes" <- w157
            "Chordnames" <- w155
            "Romans" <- w154
          }
          event "MIDI-fil": Value Change {
            w269 = 60000000  # Microseconds
            w254 = "00FF5804"  # Pre: Time Signature
            w219 = "00B07B0000FF2F00"  # End of Track
            w271 = "00FF5103"  # Pre: Set Tempo
            w274 = "4D54726B"  # Track Chunk
            w245 = "0010"  # Delta-time: ticks per quarter note
            w275 = "4D5468640000000600000001"  # Header Chunk
            # "Tracksize in bytes"
            # "Track"
            # "Note events"
            # "Collecting timesignature"
            # "Configuring the timestamp/deltatime between chords:\n4/4 gives, 4 quarternotes between each chord."
            # "Note size is given by 2^x"
            # "Meta-event setting the timesignature for the song."
            # "Timeresolution for timestamps. Set low for shorter timestamps."
            # "Meta-event setting the tempo of the song, BPM is converted in to µs per quarternote"
            # "This Event creates a MIDI-file based on the progression event and project event."
            n122 = event-data() -> ()  [unwired: 1 in, 6 out]
            n123 = local read "Project Detail"() -> (w267:T1)
            n124 = Unbundle By Name(w267) -> ("Timesignature"=w266:string)
            n125 = Concatenate Strings(w275, w245, w274) -> (w244:string)
            n126 = Hexadecimal String To Number(string=w245) -> (number=w257:u32)  [unwired: 2 in, 1 out]
            n127 = call <vilib>:"Delimited String to 1D String Array.vi"("delimiter"=" / ", "delimited string"=w266) -> ("string array"=w264:string[])  [unwired: 9 in]
            n128 = local read "Project Detail"() -> (w277:T1)
            n129 = Decimal String To Number(string=w264) -> (number=w263:i32[])  [unwired: 2 in, 1 out]
            n130 = Index Array(array=w263, index #1=0 ("index"), index #2=1 ("index")) -> (element #1=w256:i32, element #2=w252:i32)
            n131 = Unbundle By Name(w277) -> ("Bpm"=w270:i32)
            n132 = Multiply(x=4, y=w256) -> (x*y=w259:i32)
            n133 = local read "MIDI-notes"() -> (w278:string[])
            n134 = Divide(x=w259, y=w252) -> (x/y=w258:dbl)
            n135 = Logarithm Base 2(1:w252) -> (0:w250:dbl)
            n136 = Logarithm Base 2(1:2.0 ("x")) -> (0:w249:dbl)
            n137 = Divide(x=w269, y=w270) -> (x/y=w268:dbl)
            n138 = Multiply(x=w257, y=w258) -> (x*y=w216:dbl)
            n139 = Divide(x=w250, y=w249) -> (x/y=w248:dbl)
            n140 = for {
              tunnel: w278 -> [w311] mode=indexing
              shift-right: [w297] -> w276
              shift-left: "" -> [w307]
              tunnel: [w308] -> w239 mode=indexing
              tunnel: w216 -> [w305]
              n141 = call "vlq-encoder.vi"("x"=w305) -> ("Encoded Hex"=w306:u32)  [unwired: 4 in]
              n142 = call <vilib>:"Delimited String to 1D String Array.vi"("delimiter"=",", "delimited string"=w311) -> ("string array"=w309:string[])  [unwired: 9 in]
              n143 = call "vlq-encoder.vi"("x"=0) -> ("Encoded Hex"=w303:u32)  [unwired: 4 in]
              n144 = for {
                tunnel: w309 -> [w339] mode=indexing
                tunnel: [w329] -> w302 mode=indexing
                tunnel: [w330] -> w301 mode=indexing
                tunnel: w306 -> [w335]
                tunnel: w303 -> [w334]
                i -> [w337]
                w341 = "90"  # Note Off
                w340 = "00"  # Velocity
                w342 = "90"  # Note On
                # "Creating on and off events simultaneous"
                n145 = Equal To 0?(x=w337) -> (x = 0?=w336:bool)
                n146 = Select(t=w335, s=w336, f=w334) -> (s? t:f=w333:u32)
                n147 = Number To Hexadecimal String(1:i16 2 ("width (-)"), 2:w333) -> (0:w331:string)
                n148 = Concatenate Strings("00" ("string"), w342, w339, "64" ("string")) -> (w329:string)
                n149 = Concatenate Strings(w331, w341, w339, w340) -> (w330:string)
              }
              n150 = for {
                tunnel: w302 -> [w317] mode=indexing
                tunnel: w301 -> [w315] mode=indexing
                shift-right: [w316] -> w298
                shift-left: "" -> [w313]
                shift-right: [w314] -> w297
                shift-left: "" -> [w312]
                i -> [w319]
                # "Removing blanc spaces"
                n151 = Equal To 0?(x=w319) -> (x = 0?=w318:bool)
                n152 = case shown="False" w318 {
                  tunnel: w317 -> [w325 w327]
                  tunnel: [w323 w327] -> w316
                  tunnel: w315 -> [w322 w326]
                  tunnel: [w320 w326] -> w314
                  tunnel: w313 -> [w324 _]
                  tunnel: w312 -> [w321 _]
                  frame False {
                    n153 = Concatenate Strings(w324, w325) -> (w323:string)
                    n154 = Concatenate Strings(w321, w322) -> (w320:string)
                  }
                  frame True {
                  }
                }
              }
              n155 = Concatenate Strings(w307, w298) -> (w308:string)
            }
            n156 = Number To Hexadecimal String(1:i16 6 ("width (-)"), 2:w268) -> (0:w272:string)
            n157 = Number To Hexadecimal String(1:i16 2 ("width (-)"), 2:w248) -> (0:w246:string)
            n158 = Concatenate Strings(w271, w272) -> (w218:string)
            n159 = Number To Hexadecimal String(1:i16 2 ("width (-)"), 2:w256) -> (0:w253:string)
            n160 = Concatenate Strings(w254, w253, w246, "1808") -> (w217:string)
            n161 = for {
              shift-right: [w291] -> w238
              shift-left: "" -> [w289]
              tunnel: w239 -> [w290] mode=indexing
              i -> [w288]
              # "Removing blanc spaces"
              n162 = Equal To 0?(x=w288) -> (x = 0?=w292:bool)
              n163 = case shown="False" w292 {
                tunnel: [w295 w296] -> w291
                tunnel: w290 -> [w294 w296]
                tunnel: w289 -> [w293 _]
                frame False {
                  n164 = Concatenate Strings(w293, w294) -> (w295:string)
                }
                frame True {
                }
              }
            }
            n165 = Concatenate Strings(w238, w276) -> (w241:string)
            n166 = Concatenate Strings(w218, w217, w241, w219) -> (w243:string)
            n167 = String Length(string=w243) -> (length=w234:i32)
            n168 = Divide(x=w234, y=2) -> (x/y=w232:dbl)
            n169 = Number To Hexadecimal String(1:i16 8 ("width (-)"), 2:w232) -> (0:w236:string)
            n170 = Concatenate Strings(w244, w236, w243) -> (w228:string)
            n171 = String Length(string=w228) -> (length=w230:i32)
            n172 = Divide(x=w230, y=2) -> (x/y=w229:dbl)
            n173 = for {
              N: w229 -> [_]
              tunnel: [w285] -> w220 mode=indexing
              tunnel: w228 -> [w283]
              i -> [w282]
              # "Converting to bytearray"
              n174 = Multiply(x=2, y=w282) -> (x*y=w281:i32)
              n175 = String Subset(string=w283, offset (0)=w281, length (rest)=2 ("length (rest)")) -> (substring=w284:string)
              n176 = Hexadecimal String To Number(string=w284, default (0uL)=u8 0 ("default (0 U32)")) -> (number=w285:u8)  [unwired: 1 in, 1 out]
            }
            n177 = Open/Create/Replace File(prompt="Velg hvor du vil lagre MIDI-filen", operation (0:open)=T7."replace or create") -> (refnum out=w225:refnum<file>, error out=w224:errorcluster)  [unwired: 4 in, 1 out]
            n178 = Write to Binary File(file (use dialog)=w225, data=w220, error in=w224, 5:FALSE ("prepend array or string size? (T)")) -> (refnum out=w222:refnum<file>, error out=w223:errorcluster)  [unwired: 2 in, 1 out]
            n179 = Close File(refnum=w222, error in=w223) -> ()  [unwired: 2 out]
          }
          event "Guitarscale": Value Change {
            n180 = event-data() -> ()  [unwired: 1 in, 6 out]
            n181 = local read "Project Detail"() -> (w343:T1)
            n182 = local read "Notes in Scale"() -> (w344:bool[])
            n183 = call "guitarscales.vi"("Project Detail 2"=w343, "Notes in Scale in"=w344) -> ()  [unwired: 10 in]
          }
          event "Play": Value Change {
            # "This Event creates a playable loop, jamtrack, based on the progression event and project event."
            n184 = event-data() -> ()  [unwired: 1 in, 6 out]
            n185 = flat-sequence {
              tunnel: [w353] -> w350
              tunnel: [w352] -> w348
              tunnel: w350 -> [w366]
              tunnel: [w366] -> w349
              tunnel: w348 -> [w372]
              tunnel: [w372] -> w345
              tunnel: w349 -> [w374]
              tunnel: [w373] -> w346
              tunnel: w345 -> [w373]
              tunnel: [w375] -> w347
              tunnel: w346 -> [w375]
              tunnel: [w381] -> w351
              tunnel: w347 -> [w378]
              frame #0 {
                w358 = 0
                # "Initializing MIDI Out port"
                n186 = dll-call lib="/Windows/System32/winmm.dll" fn="midiOutOpen"("hmidiout"=1, "uDeviceID"=u32 0, "dwCallback"=w358, "dwCallbackInstance"=w358, "dwFlags"=w358) -> ("return type"=w356:i32, "hmidiout"=w353:i32)  [unwired: 7 in, 2 out]
                n187 = Not Equal To 0?(x=w356) -> (x != 0?=w357:bool)
                n188 = case "Error Check + Prompt" shown="True" w357 {
                  tunnel: w356 -> [_ w364]
                  tunnel: w353 -> [_ w362]
                  tunnel: [FALSE ("T button?") TRUE] -> w352
                  frame False {
                  }
                  frame True {
                    w363 = "" ("pszText")
                    # "Close MIDI out"
                    n189 = dll-call lib="/Windows/System32/winmm.dll" fn="midiOutClose"("hmidiout"=w362) -> ()  [unwired: 5 in, 2 out]
                    n190 = dll-call lib="/Windows/System32/winmm.dll" fn="midiOutGetErrorTextA"("mmrError"=w364, "pszText"=w363, "cchText"=w363) -> ("pszText"=w360:string)  [unwired: 6 in, 2 out]
                    n191 = One Button Dialog(message=w360) -> ()  [unwired: 1 in, 1 out]
                  }
                }
              }
              frame #1 {
                w368 = 0  # MIDI Ch
                # "Edit patch"
                n192 = Scale By Power Of 2(n=8, x="Instrument") -> (x*2^n=w369:i32)
                n193 = Compound Arithmetic op=ADD(w369, w368, 192) -> (w371:i32)
                n194 = dll-call lib="/Windows/System32/winmm.dll" fn="midiOutShortMsg"("hmidiout"=w366, "data"=w371) -> ()  [unwired: 6 in, 2 out]
              }
              frame #2 {
                # "Passing MIDI-handler"
                "Handler" <- w374
              }
              frame #3 {
                w376 = T8."Disabled and Grayed Out" ("Disabled")
                # "GUI config"
                n195 = property on="Create Chord Progression" class="Bool"("DisabledEnum"=w376) -> ()  [unwired: 2 in, 2 out]
                n196 = property on="Reap" class="Bool"("DisabledEnum"=w376) -> ()  [unwired: 2 in, 2 out]
                n197 = property on="Stop Music" class="Bool"("DisabledEnum"=T8."Enabled" ("Disabled")) -> ()  [unwired: 2 in, 2 out]
                n198 = property on="Exit" class="Bool"("DisabledEnum"=w376) -> ()  [unwired: 2 in, 2 out]
                n199 = property on="Play" class="Bool"("DisabledEnum"=w376) -> ()  [unwired: 2 in, 2 out]
                n200 = property on="Initiate" class="Bool"("DisabledEnum"=w376) -> ()  [unwired: 2 in, 2 out]
              }
              frame #4 {
                # "Changing State"
                n201 = Select(t=statemachine."Stop music", s=w378, f=statemachine."Play music") -> (s? t:f=w381:T6)
              }
            }
          }
        }
      }
      frame "Play music" {
        # "Sequence GUI array"
        # "Converting BPM to ms between chords"
        # "Plays generated chordprogression via MIDI, basicly the same way Windows Media Player uses MIDI-files."
        n202 = local read "Project Detail"() -> (w400:T1)
        n203 = Unbundle By Name(w400) -> ("Timesignature"=w399:string, "Bpm"=w398:i32)
        n204 = local read "MIDI-notes"() -> (w390:string[])
        n205 = local read "Handler"() -> (w391:i32)
        n206 = Divide(x=60000, y=w398) -> (x/y=w397:dbl)
        n207 = Scan From String(format string="%d / ", input string=w399, initial scan location=u32 0) -> (output 1=w396:i32)  [unwired: 2 in, 3 out]
        n208 = Array Size(array=w390) -> (size(s)=w387:i32)
        n209 = Multiply(x=w396, y=w397) -> (x*y=w392:dbl)
        n210 = Initialize Array(FALSE, w387) -> (w383:bool[])
        n211 = node-c288(w392) -> (w402:T9)  [unwired: 9 in]
        n212 = Replace Array Subset(array=w383, new element=TRUE ("new element/subarray"), index=0) -> (w382:bool[])
        n213 = timed-loop {
          timing: w402 -> [_]
          timing-out: [_] -> w401
          tunnel: w387 -> [w429]
          tunnel: ["Stop Music"] -> w389
          tunnel: w391 -> [w423]
          tunnel: w390 -> [w427]
          shift-right: [w421] -> _
          shift-left: _ -> [w417]
          tunnel: "Grunntone" -> [w409]
          tunnel: w382 -> [w408]
          i -> [w426]
          stop <- "Stop Music" stop-if-true
          n214 = node-c288() -> ()  [unwired: 1 in]
          n215 = Array Size(array=w417) -> (size(s)=w415:i32)
          n216 = Quotient & Remainder(x=w426, y=w429) -> (x-y*floor(x/y)=w407:i32)  [unwired: 1 out]
          n217 = Select(t=1, s=w409, f=w415) -> (s? t:f=w413:i32)
          n218 = Increment(x=w407) -> ()  [unwired: 1 out]
          n219 = Index Array(array=w427, index=w407) -> (element=w425:string)
          n220 = Rotate 1D Array(1:w408, 2:w407) -> (0:→"Chord active":bool[])
          n221 = call <vilib>:"Delimited String to 1D String Array.vi"("delimiter"=",", "delimited string"=w425) -> ("string array"=w420:string[])  [unwired: 9 in]
          n222 = Decimal String To Number(string=w420) -> (number=w416:i32[])  [unwired: 2 in, 1 out]
          n223 = flat-sequence {
            tunnel: w423 -> [w433]
            tunnel: [w432] -> w422
            tunnel: w416 -> [w432]
            tunnel: w417 -> [w431]
            tunnel: w413 -> [w430]
            tunnel: w423 -> [w449]
            tunnel: w422 -> [w450]
            tunnel: [w450] -> w421
            tunnel: [w448] -> w419
            tunnel: [w447] -> w418
            tunnel: w410 -> [w446]
            frame #0 {
              n224 = for {
                N: w430 -> [_]
                tunnel: w433 -> [w437]
                tunnel: w431 -> [w436] mode=indexing
                stop <- w435 stop-if-true
                w441 = 0  # MIDI Ch
                w440 = 99  # Vel
                # "Note off event"
                n225 = Scale By Power Of 2(n=16, x=w440) -> (x*2^n=w444:i32)
                n226 = Scale By Power Of 2(n=8, x=w436) -> (x*2^n=w445:i32)
                n227 = Compound Arithmetic op=ADD(w444, w445, 128, w441) -> (w438:i32)
                n228 = dll-call lib="/Windows/System32/winmm.dll" fn="midiOutShortMsg"("hmidiout"=w437, "data"=w438) -> ("return type"=w434:i32)  [unwired: 5 in, 2 out]
                n229 = Not Equal To 0?(x=w434) -> (x != 0?=w435:bool)
              }
            }
            frame #1 {
              n230 = for {
                N: w446 -> [_]
                tunnel: w450 -> [w454] mode=indexing
                tunnel: w449 -> [w453]
                tunnel: [w452] -> w448
                tunnel: [w451] -> w447
                stop <- w451 stop-if-true
                w458 = 0  # MIDI Ch
                # "Note on event"
                n231 = Scale By Power Of 2(n=16, x="Volume") -> (x*2^n=w461:i32)
                n232 = Scale By Power Of 2(n=8, x=w454) -> (x*2^n=w462:i32)
                n233 = Compound Arithmetic op=ADD(w461, w462, 144, w458) -> (w455:i32)
                n234 = dll-call lib="/Windows/System32/winmm.dll" fn="midiOutShortMsg"("hmidiout"=w453, "data"=w455) -> ("return type"=w452:i32)  [unwired: 5 in, 2 out]
                n235 = Not Equal To 0?(x=w452) -> (x != 0?=w451:bool)
              }
            }
          }
          n236 = Array Size(array=w416) -> (size(s)=w411:i32)
          n237 = Select(t=1, s=w409, f=w411) -> (s? t:f=w410:i32)
          n238 = case shown="True" w418 {
            tunnel: w419 -> [_ w463]
            frame False {
            }
            frame True {
              w464 = "" ("pszText")
              n239 = dll-call lib="/Windows/System32/winmm.dll" fn="midiOutGetErrorTextA"("mmrError"=w463, "pszText"=w464, "cchText"=w464) -> ("pszText"=w466:string)  [unwired: 6 in, 2 out]
              n240 = One Button Dialog(message=w466, button name ("OK")="Is this ok for you?") -> ()  [unwired: 1 out]
            }
          }
          n241 = node-c288() -> ()  [unwired: 1 out]
        }
        n242 = node-c288(w401) -> ()  [unwired: 7 out]
        n243 = Select(t=statemachine."Stop music", s=w389, f=statemachine."Play music") -> (s? t:f=w403:T6)
      }
      frame "Stop music" {
        # "Stops playing the Chord Progression"
        n244 = flat-sequence {
          tunnel: [w476] -> w474
          tunnel: w474 -> [w485]
          tunnel: [w485] -> w473
          tunnel: w473 -> [w488]
          tunnel: [statemachine."Wait for Event"] -> w475
          frame #0 {
            # "Turning off notes"
            n245 = local read "Handler"() -> (w476:i32)
            n246 = dll-call lib="/Windows/System32/winmm.dll" fn="midiOutReset"("hmo"=w476) -> ("return type"=w477:i32)  [unwired: 4 in, 2 out]
            n247 = Not Equal To 0?(x=w477) -> (x != 0?=w478:bool)
            n248 = case shown="True" w478 {
              tunnel: w477 -> [_ w482]
              frame False {
              }
              frame True {
                w479 = "" ("pszText")
                n249 = dll-call lib="/Windows/System32/winmm.dll" fn="midiOutGetErrorTextA"("mmrError"=w482, "pszText"=w479, "cchText"=w479) -> ("pszText"=w481:string)  [unwired: 6 in, 2 out]
                n250 = One Button Dialog(message=w481, button name ("OK")="Oks this ok for you?") -> ()  [unwired: 1 out]
              }
            }
          }
          frame #1 {
            w483 = T8."Enabled" ("Disabled")
            n251 = property on="Exit" class="Bool"("DisabledEnum"=w483) -> ()  [unwired: 2 in, 2 out]
            n252 = property on="Play" class="Bool"("DisabledEnum"=w483) -> ()  [unwired: 2 in, 2 out]
            n253 = property on="Create Chord Progression" class="Bool"("DisabledEnum"=w483) -> ()  [unwired: 2 in, 2 out]
            n254 = property on="Reap" class="Bool"("DisabledEnum"=w483) -> ()  [unwired: 2 in, 2 out]
            n255 = property on="Initiate" class="Bool"("DisabledEnum"=w483) -> ()  [unwired: 2 in, 2 out]
            n256 = property on="Stop Music" class="Bool"("DisabledEnum"=T8."Disabled and Grayed Out" ("Disabled")) -> ()  [unwired: 2 in, 2 out]
          }
          frame #2 {
            # "Closing down MIDI Out"
            n257 = dll-call lib="/Windows/System32/winmm.dll" fn="midiOutClose"("hmidiout"=w488) -> ("return type"=w486:i32)  [unwired: 4 in, 2 out]
            n258 = Not Equal To 0?(x=w486) -> (x != 0?=w487:bool)
            n259 = case shown="True" w487 {
              tunnel: w486 -> [_ w489]
              frame False {
              }
              frame True {
                w490 = "" ("pszText")
                n260 = dll-call lib="/Windows/System32/winmm.dll" fn="midiOutGetErrorTextA"("mmrError"=w489, "pszText"=w490, "cchText"=w490) -> ("pszText"=w492:string)  [unwired: 6 in, 2 out]
                n261 = One Button Dialog(message=w492, button name ("OK")="Oks this ok for you?") -> ()  [unwired: 1 out]
              }
            }
          }
          frame #3 {
            # "Changing state"
          }
        }
      }
      frame "Shut down" {
        # "Shuts down the program."
        n262 = flat-sequence {
          frame #0 {
            # "Initial shutdown"
          }
          frame #1 {
            w495 = FALSE  # Is this a simulation
            # "Shuts down program"
            n263 = case shown="False" w495 {
              frame False {
                # "Distributed version"
                n264 = Quit LabVIEW(quit? (T)=TRUE ("Is this a simulation")) -> ()
              }
              frame True {
                # "Simulation"
                n265 = Stop(stop? (T)=TRUE) -> ()
              }
            }
          }
        }
      }
      frame "MIDI-file shutdown" {
        n266 = One Button Dialog(message="MIDI-fil lagret ved Reaper prosjekt eller på ønsket plass", button name ("OK")="Ok") -> ()  [unwired: 1 out]
      }
    }
    n267 = Wait (ms)(milliseconds to wait="CPU timing") -> ()  [unwired: 1 out]
    n268 = Quotient & Remainder(x=w5, y=10) -> (x-y*floor(x/y)=→"Progression":i32)  [unwired: 1 out]
  }
